vi "ke37xx Configure Pseudocard.vi"(0 "VISA Resource Name":refnum<visa-resource-name>, 5 "Slot Number (1)":i32=1, 9 "Pseudocard Name (1: 3720)":u16(ring)=1 items=["Empty", "3720", "3721", "3722", "3723", "3724", "3730", "3731", "3740", "3750", "37320", "37321", "37322", "37323", "37324"], 11 "error in (no error)":errorcluster) -> (4 "VISA Resource Name Out":refnum<visa-resource-name>, 15 "error out":errorcluster)   [LabVIEW 2009, in "Keithley 3700 Series.lvlib"]
doc: "This VI installs a pseudocard into the DMM. A pseudocard is a virtual card which can be helpful when designing applications which use particular cards."
uses:
  <instrlib>/Keithley 3706/Keithley 3700 Series.lvlib
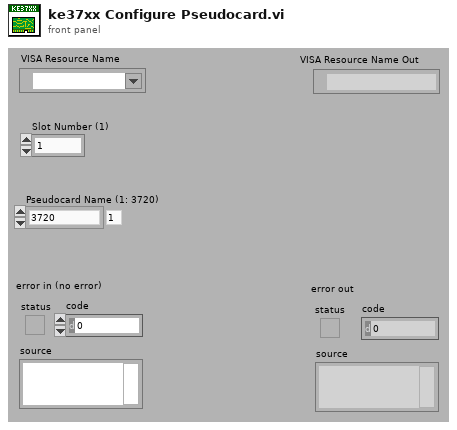
[diagram p1: front panel]
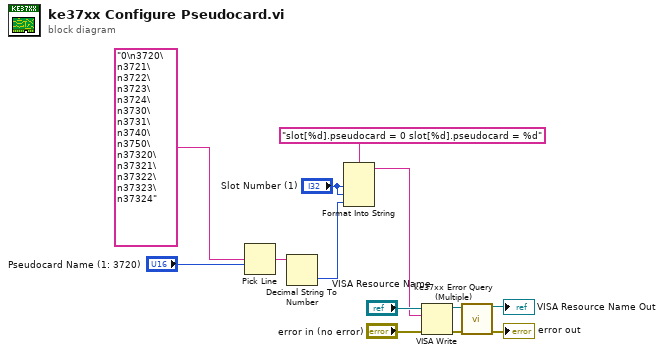
[diagram p0: block diagram]
diagram:
  n1 = Pick Line(multi-line string="0\n3720\n3721\n3722\n3723\n3724\n3730\n3731\n3740\n3750\n37320\n37321\n37322\n37323\n37324", line index="Pseudocard Name (1: 3720)") -> (output string=w3:string)  [unwired: 1 out]
  n2 = Decimal String To Number(string=w3) -> (number=w2:i32)  [unwired: 1 in, 2 out]
  n3 = Format Into String(format string="slot[%d].pseudocard = 0 slot[%d].pseudocard = %d", "Slot Number (1)", "Slot Number (1)", w2) -> (resulting string=w4:string)  [unwired: 2 in, 1 out]
  n4 = VISA Write(VISA resource name="VISA Resource Name", write buffer=w4, error in (no error)="error in (no error)") -> (VISA resource name out=w11:refnum<visa-resource-name>, error out=w10:errorcluster)  [unwired: 1 out]
  n5 = call <instrlib>:"ke37xx Error Query (Multiple).vi"("VISA resource name"=w11, "error in (no error)"=w10) -> ("VISA resource name out"=→"VISA Resource Name Out":refnum<visa-resource-name>, "error out"=→"error out":errorcluster)  [unwired: 12 out]
